vi "set_ao2.vi"() -> ()   [LabVIEW 2012]
uses:
  <vilib>/DAQmx/write.llb/DAQmx Write (Analog 1D DBL NChan 1Samp).vi
  <vilib>/DAQmx/create/channels.llb/DAQmx Create Channel (AO-Voltage-Basic).vi
  <vilib>/DAQmx/miscellaneous.llb/DAQmx Fill In Error Info.vi
panel:
  in  "V2":dbl
  in  "V1":dbl
  in  "stop":bool
  in  "Output Channel":tag="Dev4/ao0"
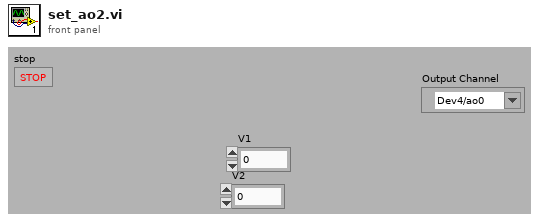
[diagram p1: front panel]
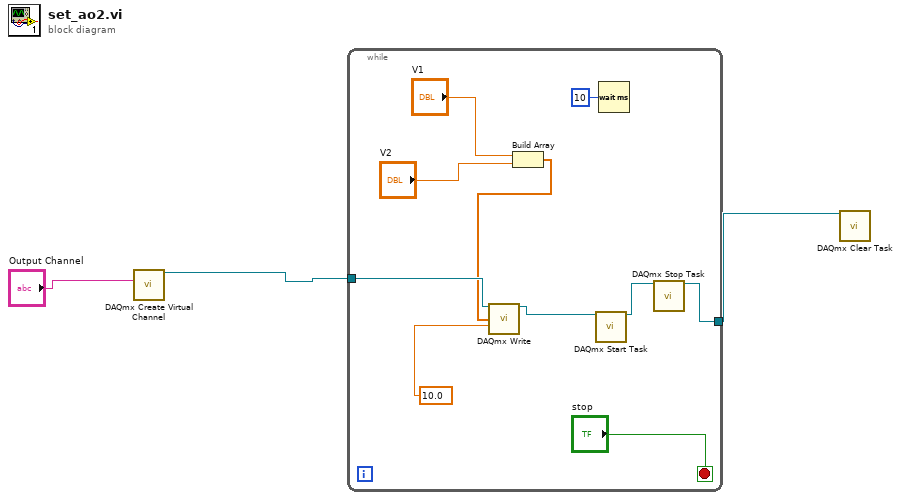
[diagram p0: block diagram]
diagram:
  n1 = call-poly <vilib>:"DAQmx Create Virtual Channel.vi"("physical channels"="Output Channel") -> ("task out"=w1:refnum<k21>)  [unwired: 8 in, 6 out]
  n2 = while {
    tunnel: [w10] -> w2
    tunnel: w1 -> [w9]
    stop <- "stop" stop-if-true
    n3 = Build Array("V1", "V2") -> (w5:dbl[])
    n4 = call-poly <vilib>:"DAQmx Write.vi"("task/channels in"=w9, "data"=w5, "timeout"=10.0) -> ("task out"=w11:refnum<k21>)  [unwired: 2 in, 10 out]
    n5 = call <vilib>:"DAQmx Start Task.vi"("task/channels in"=w11) -> ("task out"=w13:refnum<k21>)  [unwired: 1 in, 13 out]
    n6 = Wait (ms)(milliseconds to wait=u32 10) -> ()  [unwired: 1 out]
    n7 = call <vilib>:"DAQmx Stop Task.vi"("task/channels in"=w13) -> ("task out"=w10:refnum<k21>)  [unwired: 1 in, 13 out]
  }
  n8 = call <vilib>:"DAQmx Clear Task.vi"("task in"=w2) -> ()  [unwired: 1 in, 14 out]
